vi "test3.vi"() -> ()   [LabVIEW 2016]
uses:
  <vilib>/Instr/_visa.llb/VISA Configure Serial Port (Instr).vi
panel:
  out "hex integer string":string
  out "concatenated string":string
  out "Boolean":bool
  in  "Минуты":u64 max=16777215
  in  "Установка значения дв":bool
  in  "DTR Write":bool
  in  "RTS Write":bool
  in  "stop":bool
  in  "VISA resource name":refnum<visa-resource-name>
  # "1 - адресс 1 двигателя\n2 - адресс 2 двигателя\n$0MV\\01+   - запуск всех двигателей в положительном направлении \n$0MS\\00   - остановка всех двигателей\n$0MJ\\04+\\00\\00\\01   - 1 шаг всех двигателей\n$0SS\\01\\10   - скорость 10 для всех двигателей"
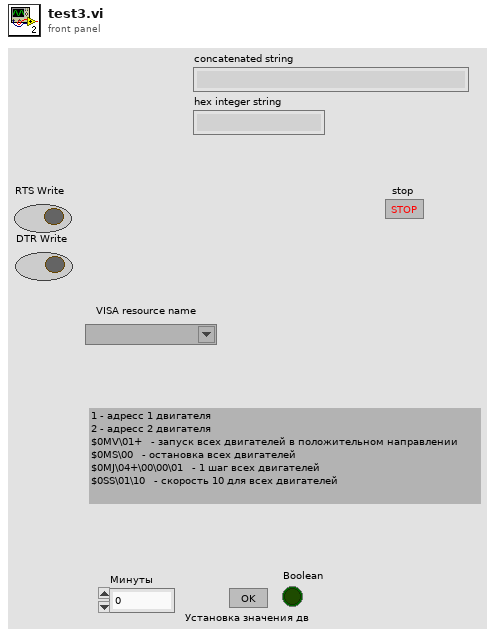
[diagram p1: front panel]
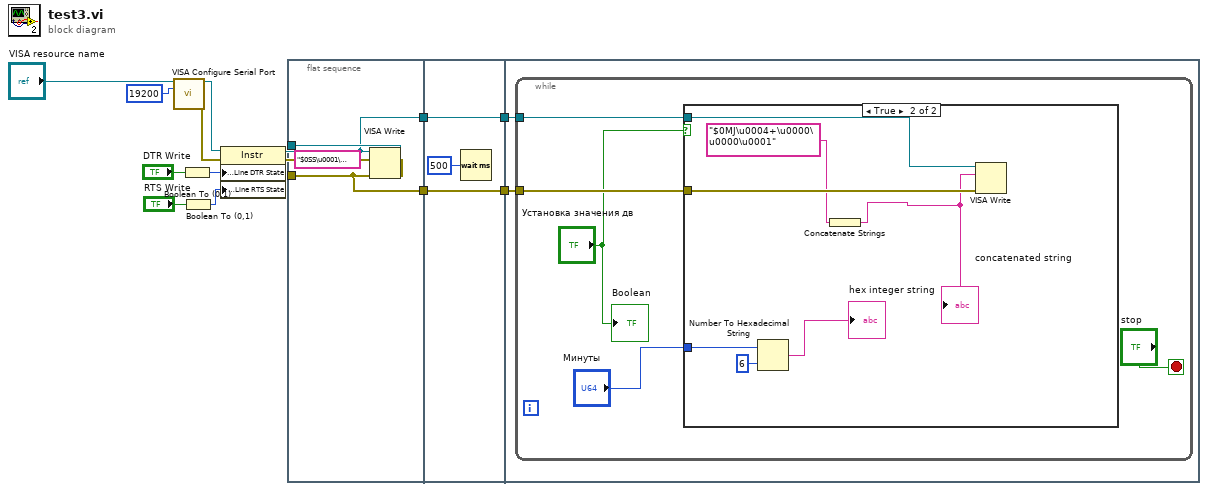
[diagram p0: block diagram]
diagram:
  n1 = call-poly "VISA Configure Serial Port"("VISA resource name"="VISA resource name", "baud rate (9600)"=u32 19200) -> ("VISA resource name out"=w8:refnum<visa-resource-name>, "error out"=w7:errorcluster)  [unwired: 12 in]
  n2 = Boolean To (0,1)(Boolean="DTR Write") -> (0, 1=w9:i16)
  n3 = Boolean To (0,1)(Boolean="RTS Write") -> (0, 1=w11:i16)
  n4 = property class="Instr"(reference=w8, error in=w7, "Serial Settings:Modem Line Settings:Line DTR State"=w9, "Serial Settings:Modem Line Settings:Line RTS State"=w11) -> (reference out=w6:refnum<visa-resource-name>, error out=w5:errorcluster)
  n5 = flat-sequence {
    tunnel: w6 -> [w16]
    tunnel: w5 -> [w15]
    tunnel: [w16] -> w3
    tunnel: [w15] -> w2
    tunnel: [w19] -> w4
    tunnel: w3 -> [w19]
    tunnel: w2 -> [w18]
    tunnel: [w18] -> w1
    tunnel: w4 -> [w22]
    tunnel: w1 -> [w21]
    frame #0 {
      n6 = VISA Write(VISA resource name=w16, write buffer="$0SS\u0001\u0010", error in (no error)=w15) -> ()  [unwired: 3 out]
    }
    frame #1 {
      n7 = Wait (ms)(milliseconds to wait=u32 500) -> ()  [unwired: 1 out]
    }
    frame #2 {
      n8 = while {
        tunnel: w22 -> [w26]
        tunnel: w21 -> [w25]
        stop <- "stop" stop-if-true
        n9 = case shown="True" "Установка значения дв" {
          tunnel: w26 -> [_ w34]
          tunnel: w25 -> [_ w33]
          tunnel: "Минуты" -> [_ w31]
          frame False {
          }
          frame True {
            n10 = Number To Hexadecimal String(1:i16 6 ("width (-)"), 2:w31) -> (0:→"hex integer string":string)
            n11 = Concatenate Strings("$0MJ\u0004+\u0000\u0000\u0001" ("write buffer")) -> (w29:string)
            "concatenated string" <- w29
            n12 = VISA Write(VISA resource name=w34, write buffer=w29, error in (no error)=w33) -> ()  [unwired: 3 out]
          }
        }
        "Boolean" <- "Установка значения дв"
      }
    }
  }
